vi "Configure Modulation (Pulse Width).vi"(0 "VISA resource name":refnum<visa-resource-name>, 1 "Enable Pulse Width Modulation (T: Enable)":bool=TRUE, 5 "Channel (0: Channel 1)":T1 items=["Channel 1", "Channel 2"], 7 "Pulse Width Modulation Source (0: Internal)":u16(ring) items=["Internal", "External"], 9 "Modulation Waveform (0: Sine)":i32(ring) items=["Sine", "Square", "Triangle", "Ramp", "Down Ramp", "Noise"], 11 "error in (no error)":errorcluster, 12 "Modulation Frequency (100.00 Hz)":dbl[unit]=100.0, 13 "Peak  Deviation (10 %)":dbl=10.0) -> (4 "VISA resource name out":refnum<visa-resource-name>, 15 "error out":errorcluster)   [LabVIEW 2009, in "Tektronix AFG 3000 Series.lvlib"]
doc: "Configures and enables pulse width modulation. The width of a pulse waveform is varied by the instantaneous voltage of the modulating waveform.\n\n<B>Note:</B>\n\nThe selected waveform must be Pulse which is configured in Configure Standard Waveform.vi for either Channel 1 or Channel 2.\n\n***NOTE: this likely doesn't correctly go back to internal if you set it to external. See \"Configure Modulation (Amplitude).vi\" for how to fix it, if needed."
uses:
  Tektronix AFG 3000 Series.lvlib
  controls.llb/Channel.ctl
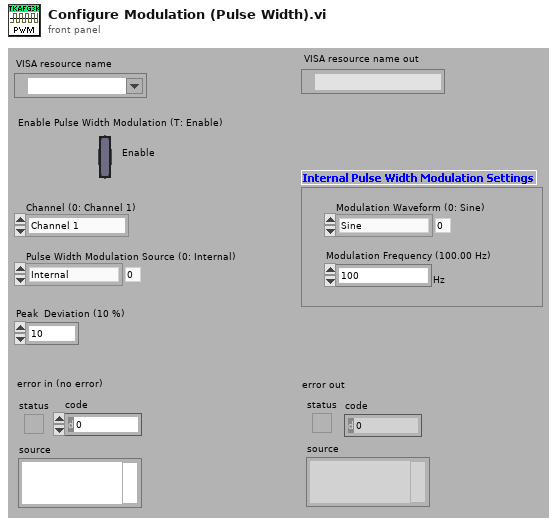
[diagram p1: front panel]
types:
  T1 = typedef "Channel.ctl" = u16
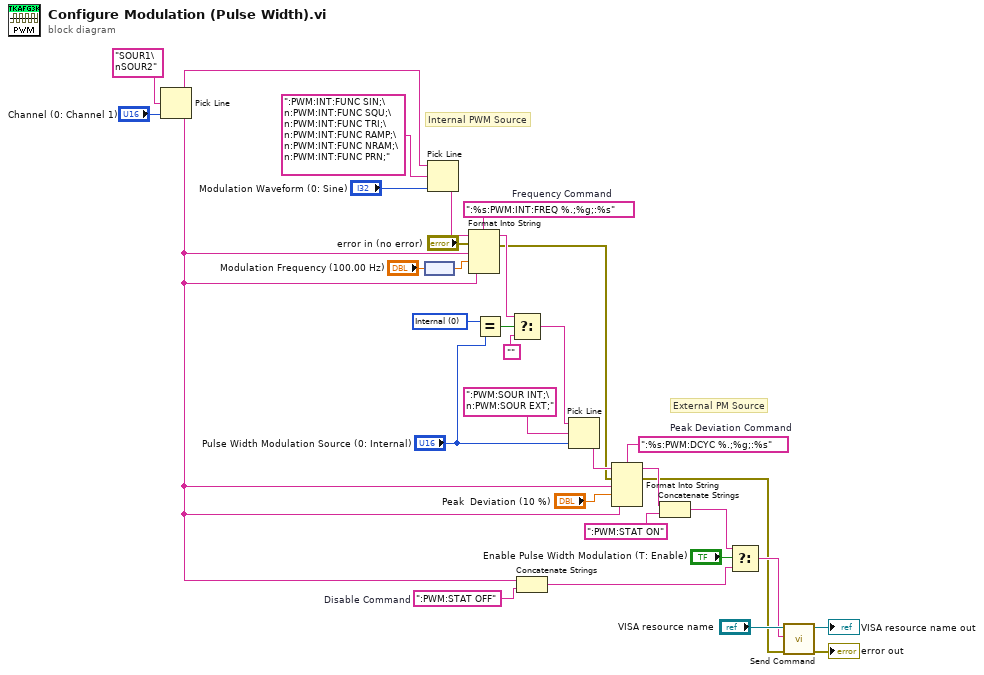
[diagram p0: block diagram]
diagram:
  w23 = ":%s:PWM:INT:FREQ %.;%g;:%s"  # Frequency Command
  w31 = ":%s:PWM:DCYC %.;%g;:%s"  # Peak Deviation Command
  w14 = u16 0 items=["Internal", "External"] ("Source (0: Internal)")
  w25 = ":PWM:STAT OFF"  # Disable Command
  # "Internal PWM Source"
  # "External PM Source"
  n1 = Pick Line(multi-line string="SOUR1\nSOUR2" ("string (\"\")"), line index="Channel (0: Channel 1)") -> (output string=w15:string)  [unwired: 1 out]
  n2 = node("Modulation Frequency (100.00 Hz)") -> (w6:dbl)
  n3 = Pick Line(string ("")=w15, multi-line string=":PWM:INT:FUNC SIN;\n:PWM:INT:FUNC SQU;\n:PWM:INT:FUNC TRI;\n:PWM:INT:FUNC RAMP;\n:PWM:INT:FUNC NRAM;\n:PWM:INT:FUNC PRN;" ("string (\"\")"), line index="Modulation Waveform (0: Sine)") -> (output string=w24:string)
  n4 = Format Into String(format string=w23, initial string=w24, error in="error in (no error)", w15, w6, w15) -> (resulting string=w18:string, error out=w8:errorcluster)
  n5 = Equal?(x=w14, y="Pulse Width Modulation Source (0: Internal)") -> (x = y?=w20:bool)
  n6 = Select(t=w18, s=w20, f="") -> (s? t:f=w12:string)
  n7 = Concatenate Strings(w15, w25) -> (w19:string)
  n8 = Pick Line(string ("")=w12, multi-line string=":PWM:SOUR INT;\n:PWM:SOUR EXT;" ("string (\"\")"), line index="Pulse Width Modulation Source (0: Internal)") -> (output string=w11:string)
  n9 = Format Into String(format string=w31, initial string=w11, error in=w8, w15, "Peak  Deviation (10 %)", w15) -> (resulting string=w29:string, error out=w1:errorcluster)
  n10 = Concatenate Strings(w29, ":PWM:STAT ON" ("Enable Command")) -> (w17:string)
  n11 = Select(t=w17, s="Enable Pulse Width Modulation (T: Enable)", f=w19) -> (s? t:f=w2:string)
  n12 = call "Send Command.vi"("error in (no error)"=w1, "write buffer"=w2, "VISA resource name"="VISA resource name") -> ("error out"=→"error out":errorcluster, "VISA resource name out"=→"VISA resource name out":refnum<visa-resource-name>)  [unwired: 7 out]
